vi "Attach.vi"(0 "reference in":refnum<class "Subject.lvclass">, 1 "ObServer.lvclass":refnum<class "ObServer.lvclass">, 5 "error in (no error)":errorcluster) -> (14 "reference out":refnum<class "Subject.lvclass">, 19 "error out":errorcluster)   [LabVIEW 2013, in "Subject.lvclass"]
uses:
  Subject.lvclass
  ObServer_class/ObServer.lvclass
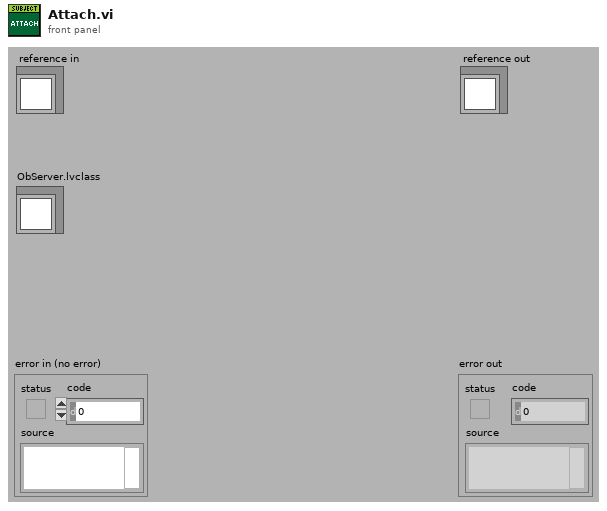
[diagram p1: front panel]
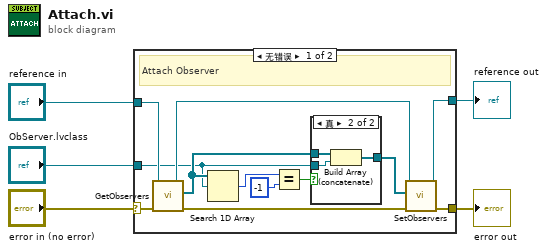
[diagram p0: block diagram]
diagram:
  n1 = case shown="无错误" "error in (no error)" {
    selector: "error in (no error)" -> [w15 w23]
    tunnel: [w6 w23] -> w4
    tunnel: [w7 w22] -> w2
    tunnel: "reference in" -> [w17 w22]
    tunnel: "ObServer.lvclass" -> [w9 _]
    frame No Error {
      # "Attach Observer"
      n2 = call-dynamic "GetObservers.vi"("error in (no error)"=w15, "reference in"=w17) -> ("error out"=w14:errorcluster, "Observers"=w10:refnum<class "ObServer.lvclass">[], "reference out"=w16:refnum<class "Subject.lvclass">)  [unwired: 7 in]
      n3 = Search 1D Array(1D array=w10, element=w9) -> (index of element=w13:i32)  [unwired: 1 in]
      n4 = Equal?(x=w13, y=-1) -> (x = y?=w11:bool)
      n5 = case shown="真" w11 {
        tunnel: w10 -> [w18 w21]
        tunnel: w9 -> [_ w20]
        tunnel: [w18 w19] -> w8
        frame False {
        }
        frame True {
          n6 = Build Array (concatenate)(w21, w20) -> (w19:refnum<class "ObServer.lvclass">[])
        }
      }
      n7 = call-dynamic "SetObservers.vi"("error in (no error)"=w14, "Observers"=w8, "reference in"=w16) -> ("error out"=w6:errorcluster, "reference out"=w7:refnum<class "Subject.lvclass">)  [unwired: 7 in]
    }
    frame Error {
    }
  }
  "error out" <- w4
  "reference out" <- w2
